vi "Shifter Toggle.vi"(8 "Pin Out":bool, 9 "Pin In":bool, 10 "Drive":bool, 11 "PTO":bool) -> (2 "Pin Status":bool, 3 "Drive/PTO":bool)   [LabVIEW 2015]
uses:
  <vilib>/ptbypt/NI_PtbyPt.lvlib
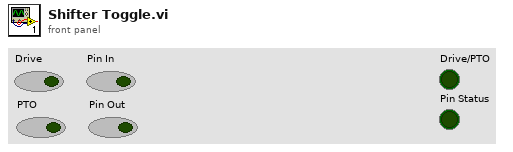
[diagram p1: front panel]
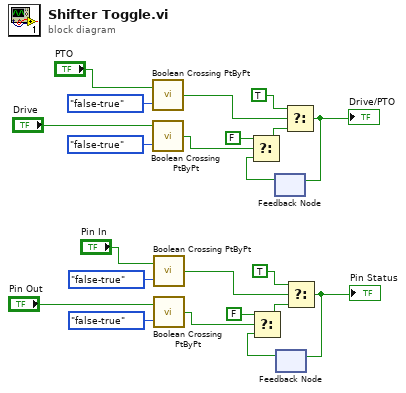
[diagram p0: block diagram]
diagram:
  n1 = call <vilib>:"Boolean Crossing PtByPt.vi"("direction"=enum16{"either", "false-true", "true-false"}."false-true", "input"="PTO") -> ("crossing"=w19:bool)  [unwired: 1 in]
  n2 = call <vilib>:"Boolean Crossing PtByPt.vi"("direction"=enum16{"either", "false-true", "true-false"}."false-true", "input"="Drive") -> ("crossing"=w20:bool)  [unwired: 1 in]
  n3 = call <vilib>:"Boolean Crossing PtByPt.vi"("direction"=enum16{"either", "false-true", "true-false"}."false-true", "input"="Pin In") -> ("crossing"=w10:bool)  [unwired: 1 in]
  n4 = call <vilib>:"Boolean Crossing PtByPt.vi"("direction"=enum16{"either", "false-true", "true-false"}."false-true", "input"="Pin Out") -> ("crossing"=w11:bool)  [unwired: 1 in]
  n5 = feedback #1() -> (w15:bool)  [unwired: 1 in]
  n6 = Select(t=FALSE, s=w20, f=w15) -> (s? t:f=w17:bool)
  n7 = feedback #2() -> (w6:bool)  [unwired: 1 in]
  n8 = Select(t=FALSE, s=w11, f=w6) -> (s? t:f=w8:bool)
  n9 = Select(t=TRUE, s=w19, f=w17) -> (s? t:f=w14:bool)
  "Drive/PTO" <- w14
  n10 = feedback-in #1(w14) -> ()
  n11 = Select(t=TRUE, s=w10, f=w8) -> (s? t:f=w5:bool)
  "Pin Status" <- w5
  n12 = feedback-in #2(w5) -> ()
